vi "Folder_exist.vi"() -> ()   [LabVIEW 2012]
panel:
  out "new_folder":path
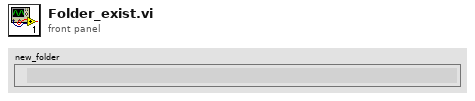
[diagram p1: front panel]
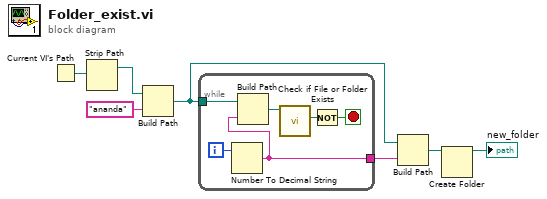
[diagram p0: block diagram]
diagram:
  n1 = Current VI's Path() -> (path=w6:path)
  n2 = Strip Path(path=w6) -> (stripped path=w5:path)  [unwired: 1 out]
  n3 = Build Path(base path=w5, name or relative path="ananda") -> (appended path=w3:path)
  n4 = while {
    tunnel: w3 -> [w13]
    tunnel: [w9] -> w4
    i -> [w12]
    stop <- w8 stop-if-true
    n5 = Number To Decimal String(number=w12) -> (decimal integer string=w9:string)  [unwired: 1 in]
    n6 = Build Path(base path=w13, name or relative path=w9) -> (appended path=w11:path)
    n7 = call <vilib>:"Check if File or Folder Exists.vi"("path"=w11) -> ("file or folder exists?"=w10:bool)  [unwired: 8 in, 2 out]
    n8 = Not(x=w10) -> (.not. x?=w8:bool)
  }
  n9 = Build Path(base path=w3, name or relative path=w4) -> (appended path=w2:path)
  n10 = Create Folder(path (use dialog)=w2) -> (created path=→"new_folder":path)  [unwired: 2 in, 2 out]
